vi "GetDataEventProperties.vi"(9 "data":T1, 10 "device name":string, 11 "data event":T5) -> (2 "data event properties":T10[](array[typedef]))   [LabVIEW 2017, in "McsaDataEventCreator.lvlib"]
uses:
  <vilib>/addons/InsightCM/Devices/Shared/Mcsa/McsaDataEventCreator/McsaDataEventCreator.lvlib
  <vilib>/addons/InsightCM/MessageBus/Base/controls/KeyValuePair.ctl
  <vilib>/addons/InsightCM/Devices/Shared/Mcsa/McsaDataEventCreator/controls/DataEventConfig.ctl
  <vilib>/addons/InsightCM/Devices/Shared/Mcsa/McsaDataEventCreator/controls/AcqParams.ctl
  <vilib>/addons/InsightCM/Devices/Shared/Common/DataAccumulator/controls/AccumulationSettings.ctl
  <vilib>/addons/InsightCM/Devices/Shared/Common/DataAccumulator/controls/accumulationType.ctl
  <vilib>/addons/InsightCM/Devices/Shared/Common/DVRBuffer/controls/BufferLocation.ctl
  <vilib>/addons/PointValueMap/controls/PointMap.ctl
  <vilib>/addons/InsightCM/Devices/Shared/Common/DataFlow/controls/Data.ctl
  <vilib>/addons/InsightCM/Utilities/DataAccessors/controls/wfmSGL_DVR.ctl
  <vilib>/addons/InsightCM/Devices/Shared/Common/DataFlow/controls/Type.ctl
  <vilib>/addons/InsightCM/Utilities/PropertyHelpers/PropertyHelpers.lvlib
  <vilib>/addons/InsightCM/Devices/Shared/Common/DataAccumulator/DataAccumulator.lvlib
  <vilib>/addons/InsightCM/Devices/Shared/Common/DVRBuffer/DVRBuffer.lvlib
  <vilib>/addons/PointValueMap/PointValueMap.lvlib
  <vilib>/addons/InsightCM/Devices/Shared/Common/DataFlow/DataFlow.lvlib
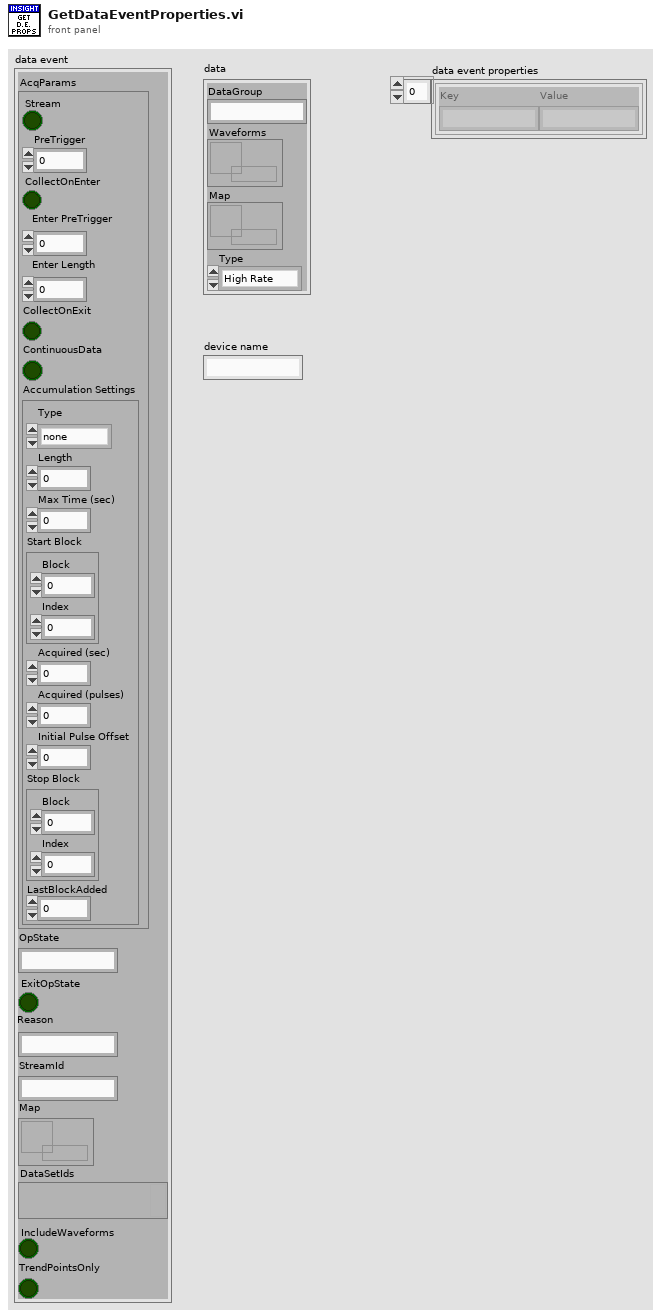
[diagram p1: front panel]
types:
  T1 = typedef "DataFlow.lvlib/Data.ctl" = cluster{"DataGroup":string, "Waveforms":T2, "Map":T3, "Type":T4}
  T2 = typedef "wfmSGL_DVR.ctl" = refnum<data-value>
  T3 = typedef "PointValueMap.lvlib/PointMap.ctl" = refnum<data-value>
  T4 = typedef "DataFlow.lvlib/Type.ctl" = enum16{"High Rate", "Low Rate", "Burst Mode"}
  T5 = typedef "McsaDataEventCreator.lvlib/DataEventConfig.ctl" = cluster{"AcqParams":T6, "OpState":string, "ExitOpState":bool, "Reason":string, "StreamId":string, "Map":T3, "DataSetIds":variant, "IncludeWaveforms":bool, "TrendPointsOnly":bool}
  T6 = typedef "McsaDataEventCreator.lvlib/AcqParams.ctl" = cluster{"Stream":bool, "PreTrigger":i32, "CollectOnEnter":bool, "Enter PreTrigger":i32, "Enter Length":dbl, "CollectOnExit":bool, "ContinuousData":bool, "Accumulation Settings":T7}
  T7 = typedef "DataAccumulator.lvlib/AccumulationSettings.ctl" = cluster{"Type":T8, "Length":dbl, "Max Time (sec)":dbl, "Start Block":T9, "Acquired (sec)":dbl, "Acquired (pulses)":i32, "Initial Pulse Offset":dbl, "Stop Block":T9, "LastBlockAdded":u32}
  T8 = typedef "DataAccumulator.lvlib/accumulationType.ctl" = enum16{"none", "seconds", "revolutions"}
  T9 = typedef "DVRBuffer.lvlib/BufferLocation.ctl" = cluster{"Block":u32, "Index":i32}
  T10 = typedef "KeyValuePair.ctl" = cluster{"Key":string, "Value":string}
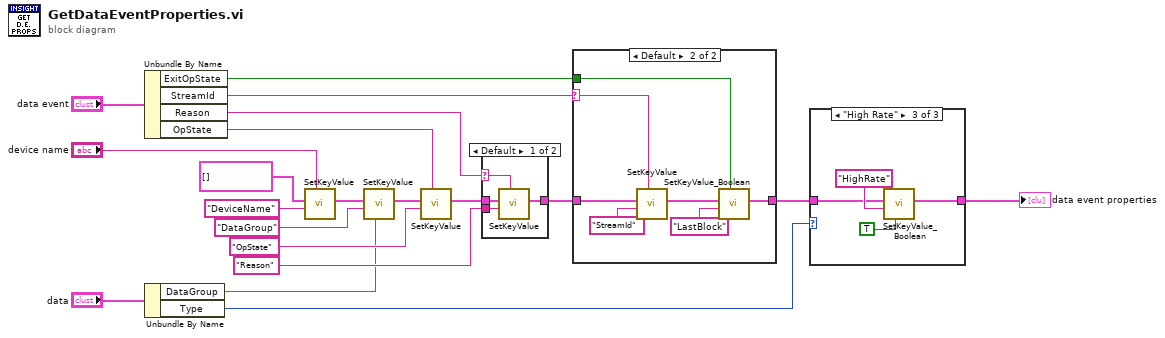
[diagram p0: block diagram]
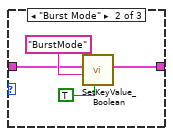
[diagram p3: hidden frame]
diagram:
  n1 = Unbundle By Name("data event") -> ("ExitOpState"=w20:bool, "StreamId"=w18:string, "Reason"=w19:string, "OpState"=w16:string)
  n2 = Unbundle By Name("data") -> ("DataGroup"=w4:string, "Type"=w2:T4)
  n3 = call <vilib>:"SetKeyValue.vi"("value"="device name", "key"="DeviceName", "key value pairs"=T10[] []) -> ("key value pairs out"=w9:T10[])  [unwired: 8 in]
  n4 = call <vilib>:"SetKeyValue.vi"("value"=w4, "key"="DataGroup", "key value pairs"=w9) -> ("key value pairs out"=w10:T10[])  [unwired: 8 in]
  n5 = call <vilib>:"SetKeyValue.vi"("value"=w16, "key"="OpState", "key value pairs"=w10) -> ("key value pairs out"=w13:T10[])  [unwired: 8 in]
  n6 = case shown="Default" w19 {
    selector: w19 -> [w21 _]
    tunnel: w13 -> [w24 w25]
    tunnel: "Reason" ("key") -> [w23 _]
    tunnel: [w22 w25] -> w17
    frame Default {
      n7 = call <vilib>:"SetKeyValue.vi"("value"=w21, "key"=w23, "key value pairs"=w24) -> ("key value pairs out"=w22:T10[])  [unwired: 8 in]
    }
    frame "" {
    }
  }
  n8 = case shown="Default" w18 {
    selector: w18 -> [_ w31]
    tunnel: w17 -> [w26 w33]
    tunnel: [w26 w29] -> w3
    tunnel: w20 -> [_ w27]
    frame "" {
    }
    frame Default {
      n9 = call <vilib>:"SetKeyValue.vi"("value"=w31, "key"="StreamId", "key value pairs"=w33) -> ("key value pairs out"=w30:T10[])  [unwired: 8 in]
      n10 = call <vilib>:"SetKeyValue_Boolean.vi"("value"=w27, "key"="LastBlock", "key value pairs"=w30) -> ("key value pairs out"=w29:T10[])  [unwired: 8 in]
    }
  }
  n11 = case shown="\"High Rate\"" w2 {
    tunnel: w3 -> [w34 w37 w41]
    tunnel: [w34 w36 w40] -> w1
    frame Default {
    }
    frame "Burst Mode" {
      n12 = call <vilib>:"SetKeyValue_Boolean.vi"("value"=TRUE, "key"="BurstMode", "key value pairs"=w37) -> ("key value pairs out"=w36:T10[])  [unwired: 8 in]
    }
    frame "High Rate" {
      n13 = call <vilib>:"SetKeyValue_Boolean.vi"("value"=TRUE, "key"="HighRate", "key value pairs"=w41) -> ("key value pairs out"=w40:T10[])  [unwired: 8 in]
    }
  }
  "data event properties" <- w1
